vi "camera_settings_to_string.vi"(8 "error in":errorcluster, 11 "Camera Setup":T1={"Analog Gain (0-5)"=4, "Frame Grabber acquisition region\n(left, top, right, bottom)"=[208, 206, 296, 279], "Exposure Time"=0.1, "EM Gain (0-255)"=175, "Trigger Polarity"="ATP P", "External Trigger Mode"="EMD E", "Scan Speed"="SSP H", "External Trigger Source"="ESC B", "Scan Mode"="SMD N", "Super Pixel Binning\n(if enabled in Scan Mode)"="SPX 1", "Camera Sub-array acquisition region\n(if enabled in scan mode)"={"Left"=0, "Top"=0, "Width"=0, "Height"=0}, "Use camera?"=FALSE, "# image buffers"=100, "Regions of Interest (Left, Top, Right, Bottom)"=[[42, 32, 50, 40]], "Background Regions (Left, Top, Right, Bottom)"=[[5, 6, 79, 17]], "shots per measurement"=100, "Photoelectron Scaling"=0.0, "Force images to U16"=FALSE} {"shots per measurement" min=0 step=1; "Background Regions (Left, Top, Right, Bottom)" min=0 max=512 step=1; "Regions of Interest (Left, Top, Right, Bottom)" min=0 max=512 step=1; "# image buffers" min=0 step=1; "Camera Sub-array acquisition region\n(if enabled in scan mode)"."Height" min=16 max=512 step=16; "Camera Sub-array acquisition region\n(if enabled in scan mode)"."Width" min=16 max=512 step=16; "Camera Sub-array acquisition region\n(if enabled in scan mode)"."Top" max=496 step=16; "Camera Sub-array acquisition region\n(if enabled in scan mode)"."Left" max=496 step=16; "Frame Grabber acquisition region\n(left, top, right, bottom)" min=0 max=512 step=1; "Analog Gain (0-5)" max=5 step=1}) -> (0 "error out":errorcluster, 3 "Camera Setup string":string)   [LabVIEW 2012]
uses:
  camera_setup.ctl
  Hamamatsu_C9100-13.lvclass
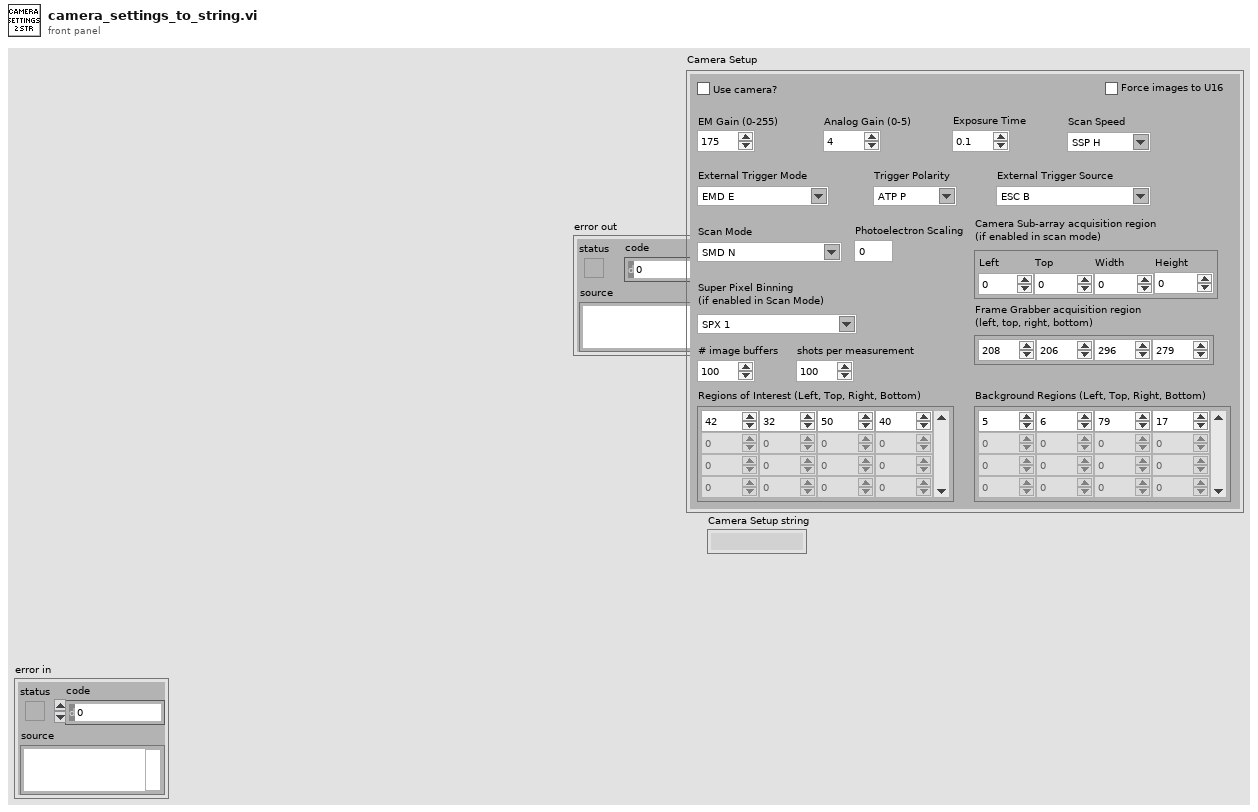
[diagram p1: front panel]
types:
  T1 = typedef "Hamamatsu_C9100-13.lvclass/camera_setup.ctl" = cluster{"Analog Gain (0-5)":u8, "Frame Grabber acquisition region\n(left, top, right, bottom)":i32[], "Exposure Time":dbl, "EM Gain (0-255)":u8, "Trigger Polarity":string, "External Trigger Mode":string, "Scan Speed":string, "External Trigger Source":string, "Scan Mode":string, "Super Pixel Binning\n(if enabled in Scan Mode)":string, "Camera Sub-array acquisition region\n(if enabled in scan mode)":cluster{"Left":u16, "Top":u16, "Width":u16, "Height":u16}, "Use camera?":bool, "# image buffers":i32, "Regions of Interest (Left, Top, Right, Bottom)":i32[][], "Background Regions (Left, Top, Right, Bottom)":i32[][], "shots per measurement":i32, "Photoelectron Scaling":dbl, "Force images to U16":bool}
  T2 = cluster{"Left":u16, "Top":u16, "Width":u16, "Height":u16}
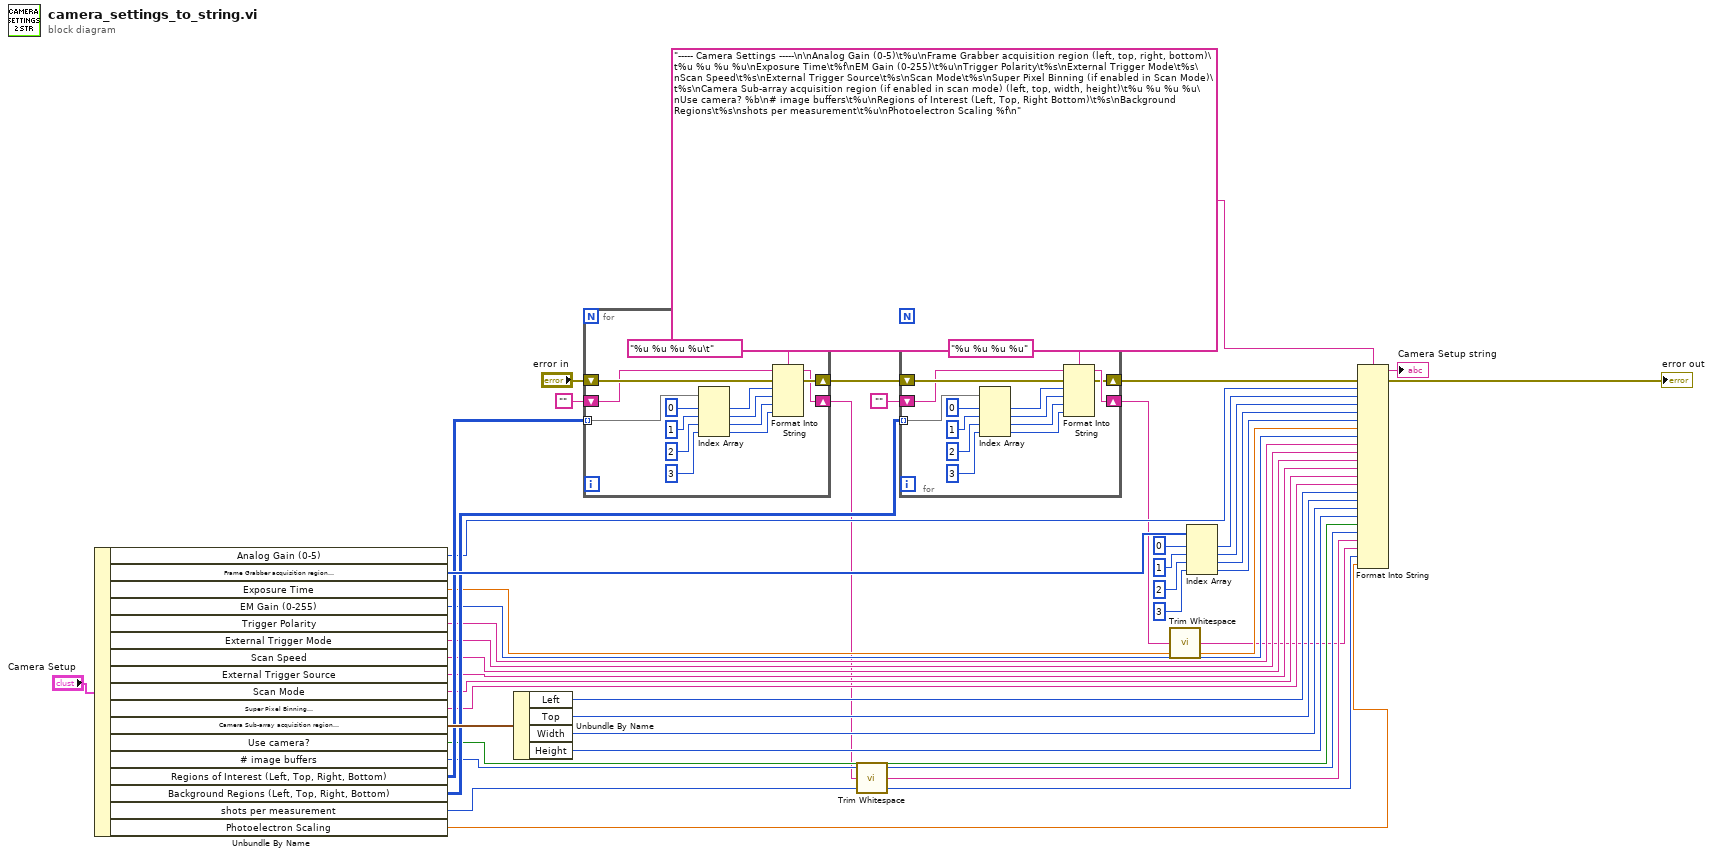
[diagram p0: block diagram]
diagram:
  n1 = Unbundle By Name("Camera Setup") -> ("Analog Gain (0-5)"=w31:u8, "Frame Grabber acquisition region\n(left, top, right, bottom)"=w42:i32[], "Exposure Time"=w25:dbl, "EM Gain (0-255)"=w24:u8, "Trigger Polarity"=w23:string, "External Trigger Mode"=w22:string, "Scan Speed"=w21:string, "External Trigger Source"=w20:string, "Scan Mode"=w19:string, "Super Pixel Binning\n(if enabled in Scan Mode)"=w18:string, "Camera Sub-array acquisition region\n(if enabled in scan mode)"=w37:T2, "Use camera?"=w13:bool, "# image buffers"=w12:i32, "Regions of Interest (Left, Top, Right, Bottom)"=w36:i32[][], "Background Regions (Left, Top, Right, Bottom)"=w35:i32[][], "shots per measurement"=w11:i32, "Photoelectron Scaling"=w1:dbl)
  n2 = Unbundle By Name(w37) -> ("Left"=w17:u16, "Top"=w16:u16, "Width"=w15:u16, "Height"=w14:u16)
  n3 = for {
    tunnel: w36 -> [w56] mode=indexing
    shift-right: [w45] -> w33
    shift-left: "error in" -> [w46]
    shift-right: [w44] -> w8
    shift-left: "" -> [w43]
    n4 = Index Array(array=w56, index #1=0 ("index"), index #2=1 ("index"), index #3=2 ("index"), index #4=3 ("index")) -> (element #1=w51:i32, element #2=w50:i32, element #3=w49:i32, element #4=w48:i32)
    n5 = Format Into String(format string="%u %u %u %u\t", initial string=w43, error in=w46, w51, w50, w49, w48) -> (resulting string=w44:string, error out=w45:errorcluster)
  }
  n6 = call <vilib>:"Trim Whitespace.vi"("string"=w8) -> ("trimmed string"=w7:string)  [unwired: 1 in]
  n7 = for {
    tunnel: w35 -> [w70] mode=indexing
    shift-right: [w58] -> w30
    shift-left: w33 -> [w59]
    shift-right: [w60] -> w5
    shift-left: "" -> [w57]
    n8 = Index Array(array=w70, index #1=0 ("index"), index #2=1 ("index"), index #3=2 ("index"), index #4=3 ("index")) -> (element #1=w65:i32, element #2=w64:i32, element #3=w63:i32, element #4=w62:i32)
    n9 = Format Into String(format string="%u %u %u %u", initial string=w57, error in=w59, w65, w64, w63, w62) -> (resulting string=w60:string, error out=w58:errorcluster)
  }
  n10 = call <vilib>:"Trim Whitespace.vi"("string"=w5) -> ("trimmed string"=w4:string)  [unwired: 1 in]
  n11 = Index Array(array=w42, index #1=0 ("index"), index #2=1 ("index"), index #3=2 ("index"), index #4=3 ("index")) -> (element #1=w29:i32, element #2=w28:i32, element #3=w27:i32, element #4=w26:i32)
  n12 = Format Into String(format string="----- Camera Settings -----\n\nAnalog Gain (0-5)\t%u\nFrame Grabber acquisition region (left, top, right, bottom)\t%u %u %u %u\nExposure Time\t%f\nEM Gain (0-255)\t%u\nTrigger Polarity\t%s\nExternal Trigger Mode\t%s\nScan Speed\t%s\nExternal Trigger Source\t%s\nScan Mode\t%s\nSuper Pixel Binning (if enabled in Scan Mode)\t%s\nCamera Sub-array acquisition region (if enabled in scan mode) (left, top, width, height)\t%u %u %u %u\nUse camera? %b\n# image buffers\t%u\nRegions of Interest (Left, Top, Right Bottom)\t%s\nBackground Regions\t%s\nshots per measurement\t%u\nPhotoelectron Scaling %f\n", error in=w30, w31, w29, w28, w27, w26, w25, w24, w23, w22, w21, w20, w19, w18, w17, w16, w15, w14, w13, w12, w7, w4, w11, w1) -> (resulting string=→"Camera Setup string":string, error out=→"error out":errorcluster)  [unwired: 1 in]
